vi "Perform Action.vi"(8 "error in":errorcluster, 10 "Input":variant, 11 "Virt Instrs FGen:Virt Waveform Generator in":refnum<class "Virt Std Waveform Generator.lvclass">) -> (0 "error out":errorcluster, 2 "Output":variant, 3 "Virt Instrs FGen:Virt Waveform Generator out":refnum<class "Virt Std Waveform Generator.lvclass">)   [LabVIEW 2023, in "Virt Instrs FGen.lvlib" / "Virt Std Waveform Generator.lvclass"]
uses:
  Virt Std Waveform Generator.lvclass
  FGen PXI/FGen PXI Std Waveform CFG/Std Waveform Action Pams.ctl
  Virt Instr Base/Virt Instr Base.lvclass/Virt Instr Base.ctl
  Virt Instr Host/Virt Instr Local.lvclass/Virt Instr Local.ctl
  Virt Std Waveform Generator.lvclass/Virt Std Waveform Generator.ctl
  Virt Instr Host/Virt Instr Local.lvclass
  Instrument/Instrument.lvclass
  FGen PXI/FGen PXI Std Waveform CFG/FGen PXI Std Waveform CFG.lvclass
  D:/git/HAL/HAL GOOP4/Virt Instr Host/Virt Instr Local.lvclass
  D:/git/HAL/HAL GOOP4/Virt Instr Base/Virt Instr Base.lvclass
  D:/git/HAL/HAL GOOP4/FGen/Virtual FGens/Virt Waveform Generator/Virt Std Waveform Generator.lvclass
  Virt Instr Base/Virt Instr Base.lvclass
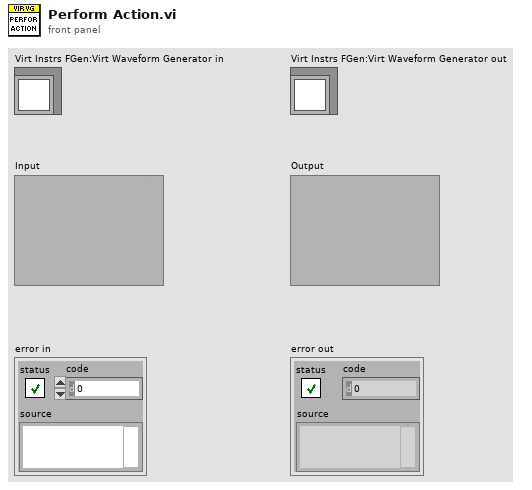
[diagram p1: front panel]
types:
  T1 = typedef "FGen PXI Std Waveform CFG.lvlib/FGen PXI Std Waveform CFG.lvclass/Std Waveform Action Pams.ctl" = cluster{"Frequency":dbl, "Amplitude":dbl, "DC Offset":dbl}
  T2 = cluster{"Channel":string, "Std Waveform Pams":T1}
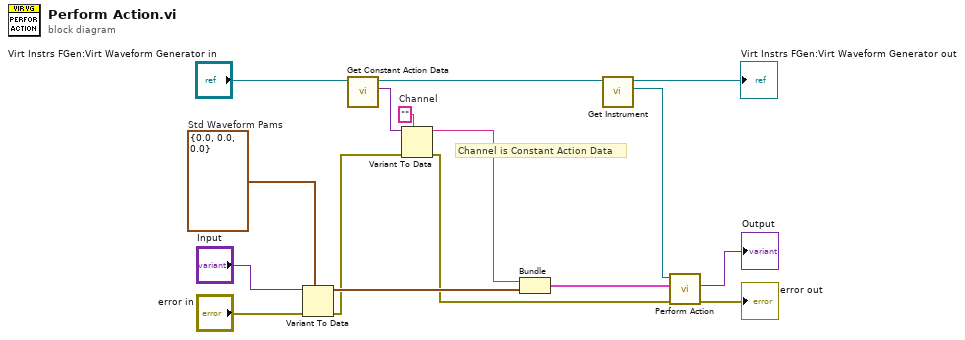
[diagram p0: block diagram]
diagram:
  w12 = ""  # Channel
  w3 = T1 {"Frequency"=0.0, "Amplitude"=0.0, "DC Offset"=0.0}  # Std Waveform Pams
  # "Channel is Constant Action Data"
  n1 = Variant To Data(error in="error in", type=w3, Variant="Input") -> (data=w14:T1, error out=w2:errorcluster)
  n2 = call "Get Constant Action Data.vi"("Virt Instr Base in"="Virt Instrs FGen:Virt Waveform Generator in") -> ("Constant Action Data"=w11:variant, "Virt Instr Base out"=w10:refnum<class "Virt Std Waveform Generator.lvclass">)  [unwired: 9 in]
  n3 = Variant To Data(error in=w2, type=w12, Variant=w11) -> (data=w5:string, error out=w1:errorcluster)
  n4 = Bundle("Channel"=w5, "Std Waveform Pams"=w14) -> (w4:T2)  [unwired: 1 in]
  n5 = call "Get Instrument.vi"("Virt Instr Base in"=w10) -> ("HAL GOOP4.lvlib:Instrument"=w9:refnum<class "Instrument.lvclass">, "Virt Instr Base out"=→"Virt Instrs FGen:Virt Waveform Generator out":refnum<class "Virt Std Waveform Generator.lvclass">)  [unwired: 9 in]
  n6 = call "Perform Action.vi"("Error In"=w1, "Input"=w4, "reference in"=w9) -> ("Error Out"=→"error out":errorcluster, "Output"=→"Output":variant)  [unwired: 6 in, 1 out]
